vi "DoCalibrationOld.vi"() -> ()   [LabVIEW 2015]
uses:
  <vilib>/Utility/file.llb/Read From Spreadsheet File (string).vi
  Desktop/Mari/GlobalData.vi
  <vilib>/Utility/file.llb/Write Delimited Spreadsheet (DBL).vi
panel:
  out "d-param-y-surveyor":dbl=76.253
  out "d-param-x-surveyor":dbl=27.888
  out "cos-phi":dbl=0.99999712
  out "sin-phi":dbl=-0.00239
  out "y-offset":dbl=60.0
  out "x-offset":dbl=24.0
  out "n":dbl
  out "appended array":dbl[][](array[numeric]) format="%.3f"
  out "Array 2":dbl[](array[numeric])
  out "Array":dbl[](array[numeric])
  out "yraw":dbl
  out "xraw":dbl
  out "Misura":string[][](table)
  out "Calib_const":string[][](table)
  out "sinT":dbl
  out "cosT":dbl
  out "ysfera":dbl format="%#.6f"
  out "xsfera":dbl format="%#_8f"
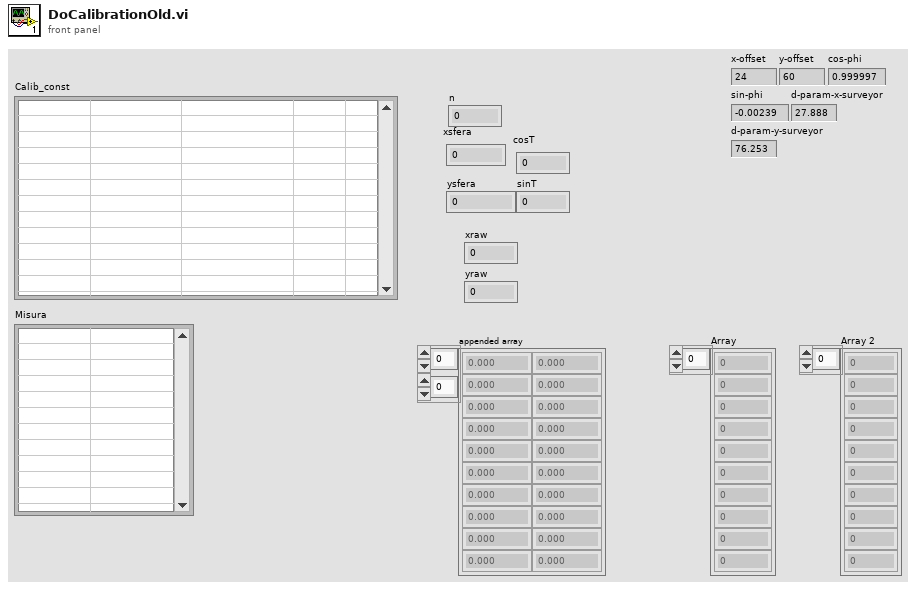
[diagram p1: front panel]
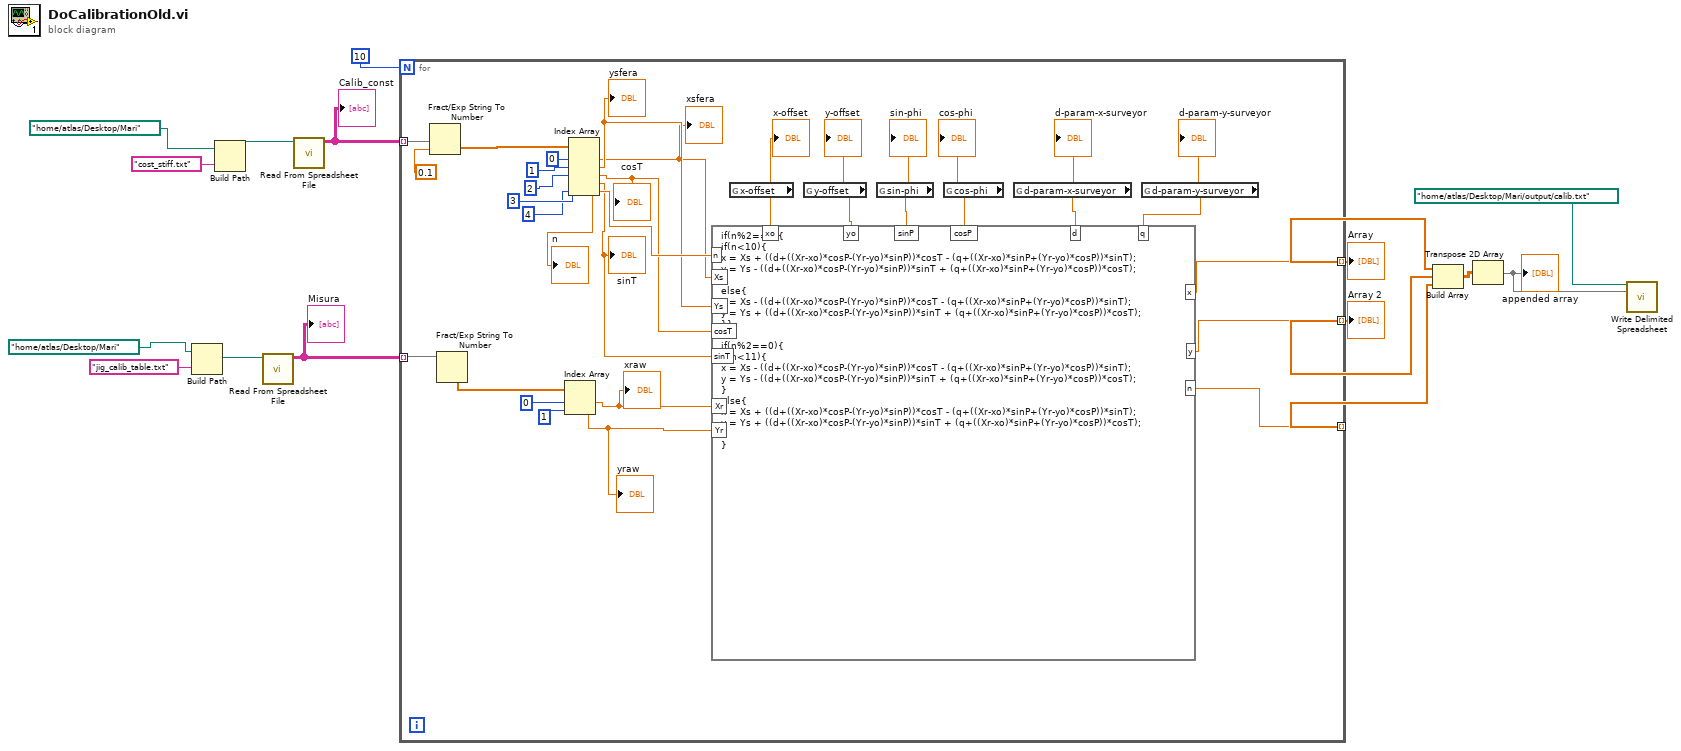
[diagram p0: block diagram]
diagram:
  n1 = Build Path(base path=path "/home/atlas/Desktop/Mari" ("file path (dialog if empty)"), name or relative path="jig_calib_table.txt") -> (appended path=w9:path)
  n2 = Build Path(base path=path "/home/atlas/Desktop/Mari" ("file path (dialog if empty)"), name or relative path="cost_stiff.txt") -> (appended path=w11:path)
  n3 = call-poly <vilib>:"Read From Spreadsheet File.vi"("file path (dialog if empty)"=w9) -> ("all rows"=w13:string[][])  [unwired: 6 in, 4 out]
  "Misura" <- w13
  n4 = call-poly <vilib>:"Read From Spreadsheet File.vi"("file path (dialog if empty)"=w11) -> ("all rows"=w14:string[][])  [unwired: 6 in, 4 out]
  "Calib_const" <- w14
  n5 = for {
    N: 10 -> [_]
    tunnel: w14 -> [w39] mode=indexing
    tunnel: w13 -> [w33] mode=indexing
    tunnel: [w32] -> w8 mode=indexing
    tunnel: [w31] -> w7 mode=indexing
    tunnel: [w22] -> w2 mode=indexing
    n6 = Fract/Exp String To Number(string=w39, default (0 dbl)=0.1 ("default (0 DBL)")) -> (number=w38:dbl[])  [unwired: 2 in, 1 out]
    n7 = Fract/Exp String To Number(string=w33) -> (number=w34:dbl[])  [unwired: 3 in, 1 out]
    n8 = Index Array(array=w34, index #1=0 ("index"), index #2=1 ("index")) -> (element #1=w23:dbl, element #2=w27:dbl)
    "xraw" <- w23
    "yraw" <- w27
    n9 = Index Array(array=w38, index #1=0 ("index"), index #2=1 ("index"), index #3=2 ("index"), index #4=3 ("index"), index #5=4 ("index")) -> (element #1=w25:dbl, element #2=w26:dbl, element #3=w28:dbl, element #4=w24:dbl, element #5=w29:dbl)
    "xsfera" <- w25
    "ysfera" <- w26
    "cosT" <- w28
    "sinT" <- w24
    "n" <- w29
    n10 = global read "GlobalData.vi" "x-offset"() -> (w21:dbl)
    "x-offset" <- w21
    n11 = global read "GlobalData.vi" "y-offset"() -> (w20:dbl)
    "y-offset" <- w20
    n12 = global read "GlobalData.vi" "sin-phi"() -> (w19:dbl)
    "sin-phi" <- w19
    n13 = global read "GlobalData.vi" "cos-phi"() -> (w18:dbl)
    "cos-phi" <- w18
    n14 = global read "GlobalData.vi" "d-param-x-surveyor"() -> (w17:dbl)
    "d-param-x-surveyor" <- w17
    n15 = global read "GlobalData.vi" "d-param-y-surveyor"() -> (w16:dbl)
    "d-param-y-surveyor" <- w16
    n16 = formula code="if(n%2==1){\nif(n<10){\nx = Xs + ((d+((Xr-xo)*cosP-(Yr-yo)*sinP))*cosT - (q+((Xr-xo)*sinP+(Yr-yo)*cosP))*sinT);\ny = Ys - ((d+((Xr-xo)*cosP-(Yr-yo)*sinP))*sinT + (q+((Xr-xo)*sinP+(Yr-yo)*cosP))*cosT);\n}\nelse{\nx = Xs - ((d+((Xr-xo)*cosP-(Yr-yo)*sinP))*cosT - (q+((Xr-xo)*sinP+(Yr-yo)*cosP))*sinT);\ny = Ys + ((d+((Xr-xo)*cosP-(Yr-yo)*sinP))*sinT + (q+((Xr-xo)*sinP+(Yr-yo)*cosP))*cosT);\n}}\n\nif(n%2==0){\nif(n<11){\nx = Xs - ((d+((Xr-xo)*cosP-(Yr-yo)*sinP))*cosT - (q+((Xr-xo)*sinP+(Yr-yo)*cosP))*sinT);\ny = Ys - ((d+((Xr-xo)*cosP-(Yr-yo)*sinP))*sinT + (q+((Xr-xo)*sinP+(Yr-yo)*cosP))*cosT);\n}\nelse{\nx = Xs + ((d+((Xr-xo)*cosP-(Yr-yo)*sinP))*cosT - (q+((Xr-xo)*sinP+(Yr-yo)*cosP))*sinT);\ny = Ys + ((d+((Xr-xo)*cosP-(Yr-yo)*sinP))*sinT + (q+((Xr-xo)*sinP+(Yr-yo)*cosP))*cosT);\n}\n}"("Xs"=w25, "sinT"=w24, "Xr"=w23, "Yr"=w27, "cosT"=w28, "Ys"=w26, "xo"=w21, "yo"=w20, "sinP"=w19, "cosP"=w18, "d"=w17, "q"=w16, "n"=w29) -> ("x"=w32:dbl, "y"=w31:dbl, "n"=w22:dbl)
  }
  "Array" <- w8
  "Array 2" <- w7
  n17 = Build Array(w8, w7, w2) -> (w6:dbl[][])
  n18 = Transpose 2D Array(2D array=w6) -> (transposed array=w5:dbl[][])
  "appended array" <- w5
  n19 = call-poly <vilib>:"Write Delimited Spreadsheet.vi"("file path (dialog if empty)"=path "/home/atlas/Desktop/Mari/output/calib.txt", "2D data"=w5) -> ()  [unwired: 12 in, 2 out]
